vi "Soln.vi"(1 "Input 2":dbl, 2 "Input 1":dbl, 3 "Operation":enum16{"Add", "Subtract", "Multiply", "Divide"}(ring)) -> (0 "Output":dbl)   [LabVIEW 2017]
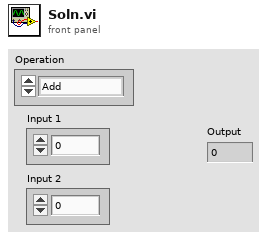
[diagram p1: front panel]
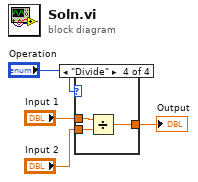
[diagram p0: block diagram]
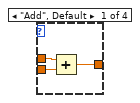
[diagram p2: hidden frame]
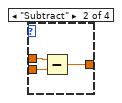
[diagram p3: hidden frame]
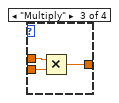
[diagram p4: hidden frame]
diagram:
  n1 = case shown="\"Divide\"" "Operation" {
    tunnel: "Input 1" -> [w7 w9 w13 w16]
    tunnel: "Input 2" -> [w6 w8 w12 w15]
    tunnel: [w5 w10 w11 w14] -> w1
    frame "Add", Default {
      n2 = Add(x=w7, y=w6) -> (x+y=w5:dbl)
    }
    frame "Subtract" {
      n3 = Subtract(x=w9, y=w8) -> (x-y=w10:dbl)
    }
    frame "Multiply" {
      n4 = Multiply(x=w13, y=w12) -> (x*y=w11:dbl)
    }
    frame "Divide" {
      n5 = Divide(x=w16, y=w15) -> (x/y=w14:dbl)
    }
  }
  "Output" <- w1
